vi "GetMotorStateByName.vi"(8 "error in (no error)":errorcluster, 10 "Channel Name":string, 11 "Motor State In":T1[](array[typedef])) -> (0 "error out":errorcluster, 1 "Motor Staste":T1, 2 "Found?":bool, 3 "Motor State Out":T1[](array[typedef]))   [LabVIEW 2016, in "McsaAnalysisFunctions.lvlib"]
uses:
  <vilib>/addons/InsightCM/Utilities/Analysis/MCSA/McsaAnalysisFunctions.lvlib
  <vilib>/addons/InsightCM/Utilities/Analysis/MCSA/controls/MotorState.ctl
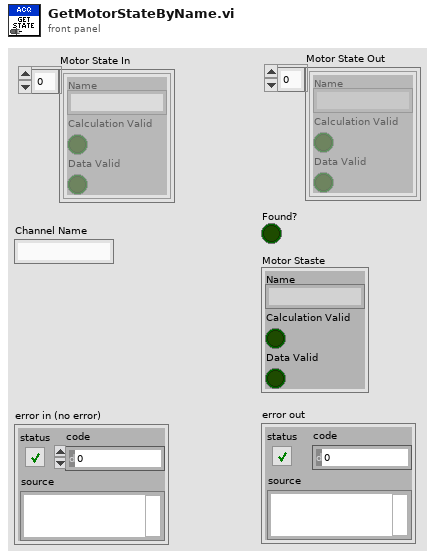
[diagram p1: front panel]
types:
  T1 = typedef "McsaAnalysisFunctions.lvlib/MotorState.ctl" = cluster{"Name":string, "Calculation Valid":bool, "Data Valid":bool}
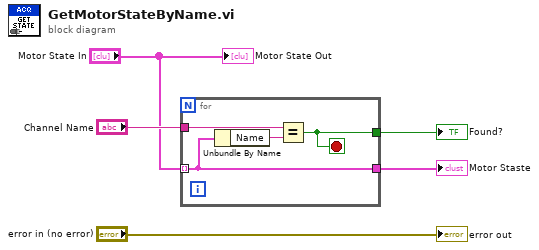
[diagram p0: block diagram]
diagram:
  n1 = for {
    tunnel: "Motor State In" -> [w7] mode=indexing
    tunnel: "Channel Name" -> [w9]
    tunnel: [w7] -> w1
    tunnel: [w8] -> w4
    stop <- w8 stop-if-true
    n2 = Unbundle By Name(w7) -> ("Name"=w6:string)
    n3 = Equal?(x=w9, y=w6) -> (x = y?=w8:bool)
  }
  "Found?" <- w4
  "Motor Staste" <- w1
  "error out" <- "error in (no error)"
  "Motor State Out" <- "Motor State In"
